vi "Configure Modulation (Pulse Width).vi"(0 "VISA resource name":refnum<visa-resource-name>, 1 "Enable Pulse Width Modulation (T: Enable)":bool=TRUE, 5 "Channel (0: Channel 1)":u16(ring) items=["Channel 1", "Channel 2"], 7 "Pulse Width Modulation Source (0: Internal)":u16(ring) items=["Internal", "External"], 9 "Modulation Waveform (0: Sine)":i32(ring) items=["Sine", "Square", "Triangle", "Ramp", "Down Ramp", "Noise", "User 1", "User 2", "User 3", "User 4", "Edit Memory"], 11 "error in (no error)":errorcluster, 12 "Modulation Frequency (100.00 Hz)":dbl=100.0, 13 "Peak  Deviation (10 %)":dbl=10.0) -> (4 "VISA resource name out":refnum<visa-resource-name>, 15 "error out":errorcluster)   [LabVIEW 2020, in "AWG.lvlib" / "Tektronix AFG 3000 Series.lvlib"]
doc: "Configures and enables pulse width modulation. The width of a pulse waveform is varied by the instantaneous voltage of the modulating waveform.\n\n<B>Note:</B>\n\nThe selected waveform must be Pulse which is configured in Configure Standard Waveform.vi for either Channel 1 or Channel 2."
uses:
  Tektronix AFG 3000 Series.lvlib
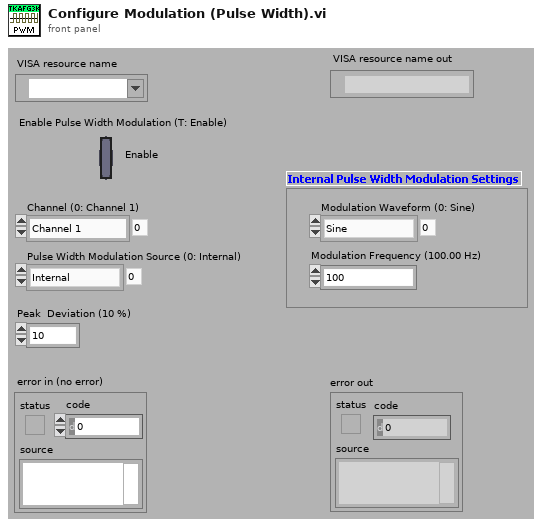
[diagram p1: front panel]
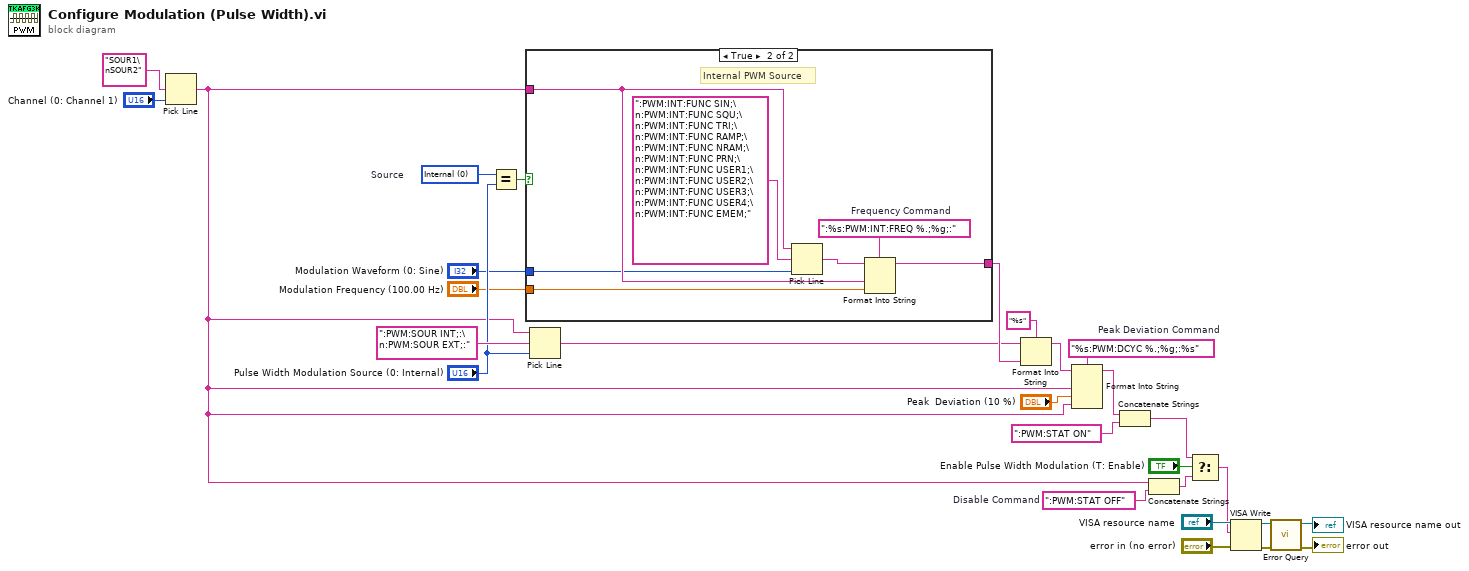
[diagram p0: block diagram]
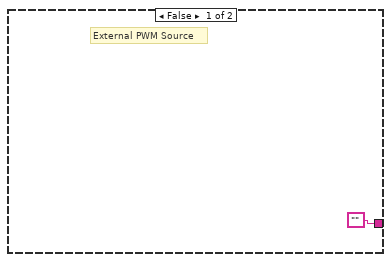
[diagram p2: hidden frame]
diagram:
  w21 = "%s:PWM:DCYC %.;%g;:%s"  # Peak Deviation Command
  w11 = u16 0 items=["Internal", "External"]  # Source
  w15 = ":PWM:STAT OFF"  # Disable Command
  n1 = Pick Line(multi-line string="SOUR1\nSOUR2" ("string (\"\")"), line index="Channel (0: Channel 1)") -> (output string=w3:string)  [unwired: 1 in]
  n2 = Equal?(x=w11, y="Pulse Width Modulation Source (0: Internal)") -> (x = y?=w9:bool)
  n3 = case shown="True" w9 {
    tunnel: ["" w33] -> w7
    tunnel: w3 -> [_ w32]
    tunnel: "Modulation Waveform (0: Sine)" -> [_ w31]
    tunnel: "Modulation Frequency (100.00 Hz)" -> [_ w30]
    frame False {
      # "External PWM Source"
    }
    frame True {
      w35 = ":%s:PWM:INT:FREQ %.;%g;:"  # Frequency Command
      # "Internal PWM Source"
      n4 = Pick Line(string ("")=w32, multi-line string=":PWM:INT:FUNC SIN;\n:PWM:INT:FUNC SQU;\n:PWM:INT:FUNC TRI;\n:PWM:INT:FUNC RAMP;\n:PWM:INT:FUNC NRAM;\n:PWM:INT:FUNC PRN;\n:PWM:INT:FUNC USER1;\n:PWM:INT:FUNC USER2;\n:PWM:INT:FUNC USER3;\n:PWM:INT:FUNC USER4;\n:PWM:INT:FUNC EMEM;" ("string (\"\")"), line index=w31) -> (output string=w36:string)
      n5 = Format Into String(format string=w35, initial string=w36, w32, w30) -> (resulting string=w33:string)  [unwired: 1 in, 1 out]
    }
  }
  n6 = Pick Line(string ("")=w3, multi-line string=":PWM:SOUR INT;:\n:PWM:SOUR EXT;:" ("string (\"\")"), line index="Pulse Width Modulation Source (0: Internal)") -> (output string=w6:string)
  n7 = Format Into String(format string="%s", initial string=w6, w7) -> (resulting string=w5:string)  [unwired: 1 in, 1 out]
  n8 = Format Into String(format string=w21, initial string=w5, w3, "Peak  Deviation (10 %)", w3) -> (resulting string=w19:string)  [unwired: 1 in, 1 out]
  n9 = Concatenate Strings(w19, ":PWM:STAT ON" ("Enable Command")) -> (w13:string)
  n10 = Concatenate Strings(w3, w15) -> (w14:string)
  n11 = Select(t=w13, s="Enable Pulse Width Modulation (T: Enable)", f=w14) -> (s? t:f=w12:string)
  n12 = VISA Write(VISA resource name="VISA resource name", write buffer=w12, error in (no error)="error in (no error)") -> (VISA resource name out=w27:refnum<visa-resource-name>, error out=w28:errorcluster)  [unwired: 1 out]
  n13 = call "Error Query.vi"("error in (no error)"=w28, "VISA resource name"=w27) -> ("error out"=→"error out":errorcluster, "VISA resource name out"=→"VISA resource name out":refnum<visa-resource-name>)  [unwired: 6 in, 2 out]
